vi "Somas subtraction.vi"(9 "Enabled? (T)":bool=TRUE, 11 "Input image (binary)":T1) -> (1 "Exposed somas":T1(plugin-control), 3 "somas subtracted":T1(plugin-control))   [LabVIEW 2017]
uses:
  <vilib>/vision/Image Controls.llb/IMAQ Image.ctl
  <vilib>/vision/NI_Vision_Development_Module.lvlib
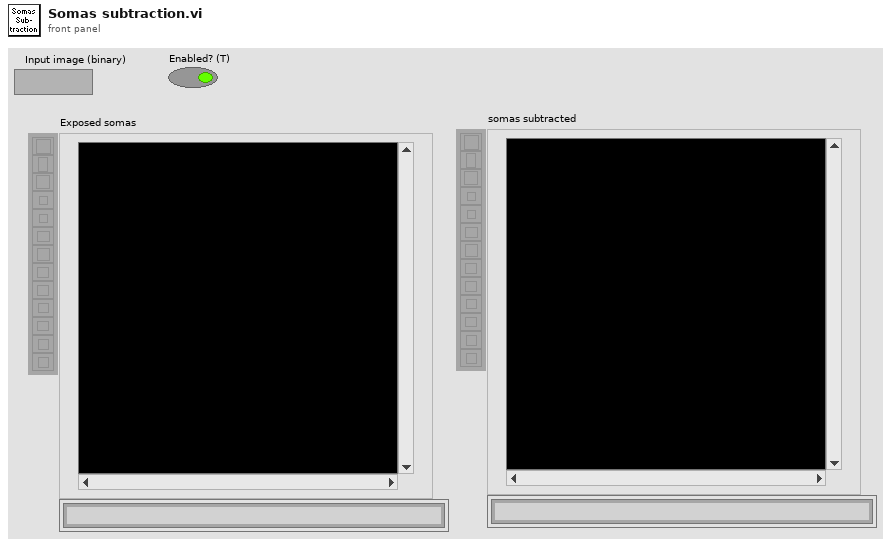
[diagram p1: front panel]
types:
  T1 = typedef "IMAQ Image.ctl" = refnum<image>
  T2 = typedef "Image Type" = u32
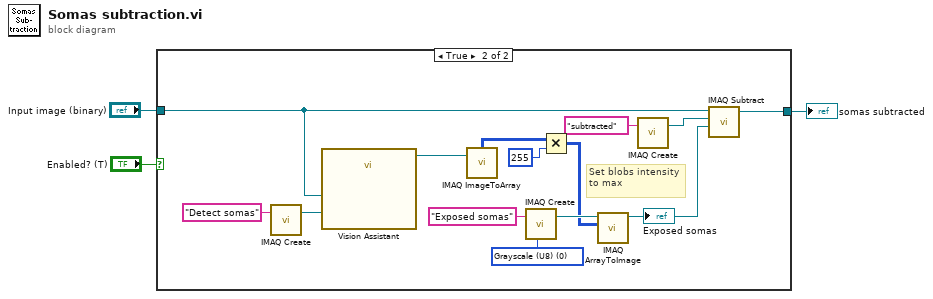
[diagram p0: block diagram]
diagram:
  n1 = case shown="True" "Enabled? (T)" {
    tunnel: [w4 w18] -> w3
    tunnel: "Input image (binary)" -> [w4 w9]
    frame False {
    }
    frame True {
      w15 = T2 0 items=["Grayscale (U8)", "Grayscale (I16)", "Grayscale (SGL)", "Complex (CSG)", "RGB (U32)", "HSL (U32)", "RGB (U64)", "Grayscale (U16)"] ("Image Type")
      # "Set blobs intensity to max"
      n2 = call "IMAQ Create"("Image Name"="Detect somas") -> ("New Image"=w6:T1)  [unwired: 4 in, 1 out]
      n3 = call "Vision Assistant"("Image In"=w9, "Image Dst"=w6) -> ("Image Out"=w11:T1)  [unwired: 24 in, 1 out]
      n4 = call "IMAQ ImageToArray"("Image"=w11) -> ("Image Pixels (U8)"=w16:u8[][])  [unwired: 3 in, 4 out]
      n5 = call "IMAQ Create"("Image Name"="Exposed somas", "Image Type"=w15) -> ("New Image"=w14:T1)  [unwired: 3 in, 1 out]
      n6 = Multiply(x=w16, y=255) -> (x*y=w13:i32[][])
      n7 = call "IMAQ ArrayToImage"("Image Pixels (U8)"=w13, "Image"=w14) -> ("Image Out"=w17:T1)  [unwired: 8 in, 1 out]
      "Exposed somas" <- w17
      n8 = call "IMAQ Create"("Image Name"="subtracted") -> ("New Image"=w8:T1)  [unwired: 4 in, 1 out]
      n9 = call "IMAQ Subtract"("Image Src A"=w9, "Image Dst"=w8, "Image Src B"=w17) -> ("Image Dst Out"=w18:T1)  [unwired: 4 in, 1 out]
    }
  }
  "somas subtracted" <- w3
